vi "Test U8 Subscriber.vi"() -> ()   [LabVIEW 2021]
uses:
  ChannelCommon/typedef/FIFO Config.ctl
  ChannelCommon/ChannelCommon.lvlib
  CIFChannels/Typedef/Direction.ctl
  CIFChannels/CIFChannels.lvclass
  CIF_CIPC_Fifo_DAQ.lvclass
panel:
  in  "millisecond multiple":u32
  out "U8 Data":u8[](array[numeric])
  in  "stop":bool
  out "timed out?":bool
  out "error out":errorcluster
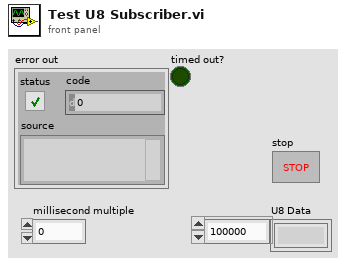
[diagram p1: front panel]
types:
  T1 = typedef "ChannelCommon.lvlib/FIFO Config.ctl" = cluster{"Max Bytes/Msg":u64, "Max Msg/FIFO":u64, "Flags":u64}
  T2 = typedef "CIFChannels.lvclass/Direction.ctl" = enum16{"Publisher", "Subscriber"}
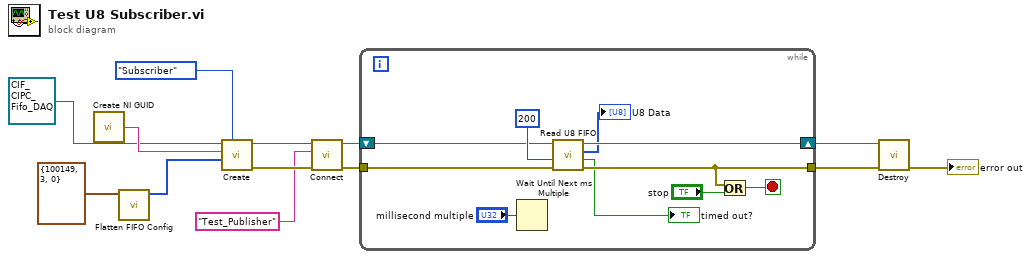
[diagram p0: block diagram]
diagram:
  n1 = call <vilib>:"Create NI GUID.vi"() -> ("NI GUID"=w8:string)
  n2 = call "Flatten FIFO Config.vi"("FIFO Config in"=T1 {"Max Bytes/Msg"=100149, "Max Msg/FIFO"=3, "Flags"=0}) -> ("Flattened FIFO Config"=w2:u8[])  [unwired: 10 in]
  n3 = call-dynamic "Create.vi"("Direction"=Direction."Subscriber", "Custom Config Data"=w2, "Name"=w8, "CIFFIFO in"=refnum<class "CIF_CIPC_Fifo_DAQ.lvclass"> refnum ("CIF_CIPC_Fifo_U8.lvclass")) -> ("error out"=w10:errorcluster, "CIFFIFO out"=w11:refnum<class "CIF_CIPC_Fifo_DAQ.lvclass">)  [unwired: 6 in]
  n4 = call-dynamic "Connect.vi"("error in (no error)"=w10, "Connection Name"="Test_Publisher", "CIFTag in"=w11) -> ("error out"=w4:errorcluster, "CIFTag out"=w7:refnum<class "CIF_CIPC_Fifo_DAQ.lvclass">)  [unwired: 7 in]
  n5 = while {
    shift-right: [w23] -> w13
    shift-left: w7 -> [w21]
    tunnel: w4 -> [w20]
    tunnel: [w17] -> w3
    stop <- w15 stop-if-true
    n6 = Wait Until Next ms Multiple(millisecond multiple="millisecond multiple") -> ()  [unwired: 1 out]
    n7 = call-dynamic "Read U8 FIFO.vi"("error in (no error)"=w20, "Timeout (ms)"=200, "CIFFIFO in"=w21) -> ("error out"=w17:errorcluster, "timed out?"=→"timed out?":bool, "Data out"=→"U8 Data":u8[], "CIFFIFO out"=w23:refnum<class "CIF_CIPC_Fifo_DAQ.lvclass">)  [unwired: 4 in, 1 out]
    n8 = Or(x=w17, y="stop") -> (x .or. y?=w15:bool)
  }
  n9 = call-dynamic "Destroy.vi"("error in (no error)"=w3, "CIFTag in"=w13) -> ("error out"=→"error out":errorcluster)  [unwired: 8 in, 1 out]
